vi "Measurement on Remote PC.vi"(3 "Mode":T5, 5 "Traverse line In":T1 {"Carrier_2 Q (l/min)" format="%#.2f"; "Row Duration (mins)" format="%#.1f"; "Row No" min=0; "Trace Gas Concentration (%)" min=0.0 format="%#_4f"; "Carrier_1 Q (l/min)" format="%#.4f"; "Start X" format="%#.2f"; "Start Y" format="%#.2f"; "Start Z" format="%#.2f"; "End X" format="%#.2f"; "End Y" format="%#.2f"; "End Z" format="%#.2f"; "Tunnel Speed" format="%#.2f"; "Averaging time (mins)" min=0.0 format="%#.2f"}) -> (0 "Error Message":string, 1 "Status":T4, 2 "Traverse line Out":T1 {"Carrier_2 Q (l/min)" format="%#.2f"; "Row Duration (mins)" format="%#.1f"; "Row No" min=0; "Trace Gas Concentration (%)" min=0.0 format="%#_4f"; "Carrier_1 Q (l/min)" format="%#.4f"; "Start X" format="%#.2f"; "Start Y" format="%#.2f"; "Start Z" format="%#.2f"; "End X" format="%#.2f"; "End Y" format="%#.2f"; "End Z" format="%#.2f"; "Tunnel Speed" format="%#.2f"; "Averaging time (mins)" min=0.0 format="%#.2f"})   [LabVIEW 2020]
uses:
  Gen Trav/Traverse_cluster.ctl
  Gen Trav/Spacing.ctl
  Controls/Multi_run_mode.ctl
  Controls/User_Specific_mode.ctl
  Gen Trav/Multi_Run_Status.ctl
  Controls/Save_Data.ctl
  Controls/Setup.ctl
panel:
  # "X           Y          Z"
  # "Start"
  # "End"
  # "X           Y          Z"
  # "Start"
  # "End"
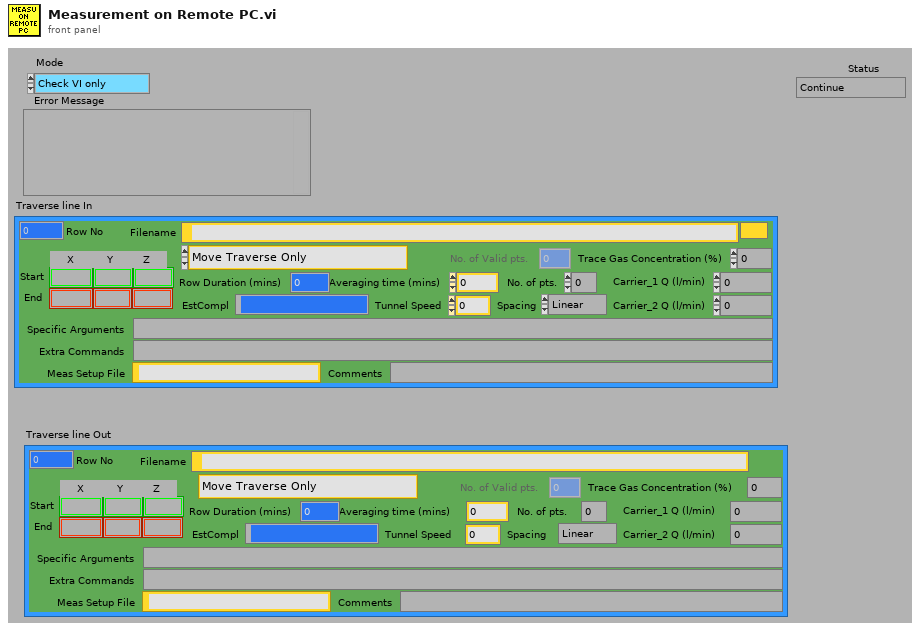
[diagram p1: front panel]
types:
  T1 = typedef "Traverse_cluster.ctl" = cluster{"Start X":sgl, "Start Y":sgl, "Start Z":sgl, "End X":sgl, "End Y":sgl, "End Z":sgl, "No. of pts.":i32, "Spacing":T2, "Filename":path, "Tunnel Speed":dbl, "Averaging time (mins)":dbl, "Extra Commands":string, "Carrier_1 Q (l/min)":dbl, "Carrier_2 Q (l/min)":dbl, "Trace Gas Concentration (%)":dbl, "Specific Arguments":string, "Comments":string, "Row No":i32, "Row Type Selector":T3, "EstCompl":string, "Row Duration (mins)":dbl, "No. of Valid pts.":i32, "Meas Setup File":string}
  T2 = typedef "Spacing.ctl" = enum16{"Linear", "Log", "Gauss", "Specified", "N/A"}
  T3 = typedef "Multi_run_mode.ctl" = enum16{"Move Traverse Only", "Set Tunnel Speed Only", "Set Source Only", "Set Measurement Conditions", "Single Measurement", "Vertical Profile", "Lateral Profile", "Longitudinal Profile", "Multi-Axis Profile", "Explore Volume", "Auto Calibrate", "Meas Fast FID Bkgnd", "Check Beam Power", "Scanning Valve Measurement", "Run VI Named:", "Set ADAM Ch", "Wait (minutes)", "Send Message", "Synchronize With:", "Fall Back to this Row", "Turn Off Row Repeating", "Traverse 3D Volume", "Blank Row", "Jump to Fall Back Row"}
  T4 = typedef "Multi_Run_Status.ctl" = enum16{"Continue", "Continue with Error", "Jump to Next Point", "Jump to Next Row", "Jump To Fall Back", "Terminate Run"}
  T5 = typedef "User_Specific_mode.ctl" = enum16{"Check VI only", "Run VI"}
  T6 = typedef "Status_Cluster.ctl" = cluster{"Status":T4, "Error Type":string, "Error Description":string}
  T7 = typedef "Setup.ctl" = enum16{"Run Program", "Show Setup", "Save Current Setup", "Setup Front Panel"}
  T8 = typedef "Save_Data.ctl" = enum16{"Save No Data", "Save Data"}
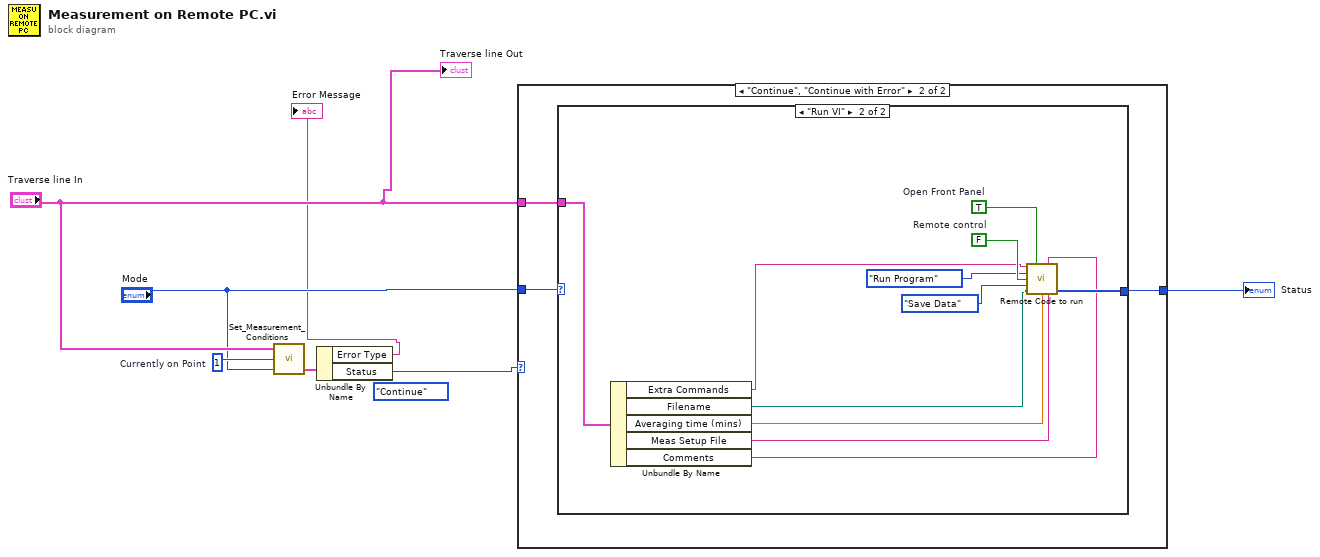
[diagram p0: block diagram]
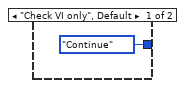
[diagram p3: hidden frame]
diagram:
  (unwired) Multi_Run_Status."Continue" ("Status")
  w5 = 1  # Currently on Point
  n1 = call "Set_Measurement_Conditions.vi"("Simulate/Run"="Mode", "Currently on Point"=w5, "Traverse line"="Traverse line In") -> ("Status Cluster"=w6:T6)  [unwired: 2 out]
  n2 = Unbundle By Name(w6) -> ("Error Type"=→"Error Message":string, "Status"=w1:T4)
  n3 = case shown="\"Continue\", \"Continue with Error\"" w1 {
    selector: w1 -> [w8 _]
    tunnel: [w8 w11] -> w7
    tunnel: "Traverse line In" -> [_ w10]
    tunnel: "Mode" -> [_ w9]
    frame Default {
    }
    frame "Continue", "Continue with Error" {
      n4 = case shown="\"Run VI\"" w9 {
        tunnel: [Multi_Run_Status."Continue" ("Status") w20] -> w11
        tunnel: w10 -> [_ w19]
        frame "Check VI only", Default {
        }
        frame "Run VI" {
          w21 = TRUE  # Open Front Panel
          w23 = FALSE  # Remote control
          n5 = Unbundle By Name(w19) -> ("Extra Commands"=w15:string, "Filename"=w16:path, "Averaging time (mins)"=w22:dbl, "Meas Setup File"=w14:string, "Comments"=w13:string)
          n6 = call "Remote Code to run.vi"("Extra command String"=w15, "Open Front Panel"=w21, "Current Row Comments"=w13, "setup"=Setup."Run Program", "Remote control"=w23, "File"=Save_Data."Save Data", "Results Filename"=w16, "Averaging time (min)"=w22, "Setup filename"=w14) -> ("Status"=w20:T4)  [unwired: 6 in]
        }
      }
    }
  }
  "Status" <- w7
  "Traverse line Out" <- "Traverse line In"
